vi "Main_copy.vi"(0 "PID On":bool) -> (5 "Total (V)":dbl[](array[slide]) scale=-8.0..8.0, 6 "Force (N)":T3(graph)={"M1 ref force"=20.0, "M2 ref force"=10.768311870905725, "M1 mes force"=3.690819426740976, "M2 mes force"=4.004504201458466})   [LabVIEW 2021]
uses:
  <vilib>/Platform/TimedLoop/XDataNode/timing_clust.ctl
  <vilib>/Platform/TimedLoop/XDataNode/nitl_modes.ctl
  <vilib>/Platform/TimedLoop/XDataNode/wakeup.ctl
  <vilib>/DAQmx/write.llb/DAQmx Write (Digital 1D Bool 1Chan 1Samp).vi
  <vilib>/DAQmx/write.llb/DAQmx Write (Analog 1D DBL NChan 1Samp).vi
  <vilib>/DAQmx/create/channels.llb/DAQmx Create Channel (DO-Digital Output).vi
  <vilib>/DAQmx/create/channels.llb/DAQmx Create Channel (AO-Voltage-Basic).vi
  <vilib>/DAQmx/create/channels.llb/DAQmx Create Channel (AI-Voltage-Basic).vi
  <vilib>/addons/control/pid/pid.llb/PID (DBL).vi
  <vilib>/DAQmx/miscellaneous.llb/DAQmx Fill In Error Info.vi
  <vilib>/Platform/TimedLoop/XDataNode/XDataNode.xnode
  <vilib>/Platform/TimedLoop/XDataNode/XDNodeRunTimeDep.lvlib
  <vilib>/addons/control/pid/NI_PID_pid.lvlib
panel:
  out "Control Time (ms)":i32
  out "Real Time (ms)":u32
  in  "RBF":bool
  in  "Traj Start":bool
  in  "PID gains":T1={"proportional gain (Kc)"=0.15, "integral time (Ti, min)"=0.0, "derivative time (Td, min)"=0.0} {"derivative time (Td, min)" format="%.3f"; "integral time (Ti, min)" format="%.3f"; "proportional gain (Kc)" format="%.3f"}
  out "output":dbl(slide)=-9.231688129094275 scale=-40.0..40.0
  in  "Set Tension":dbl=3.0
  in  "PID Tab":enum32{"PID Gain", "PIN On"}(tab)=enum."PIN On"
  in  "Gains":T2(array[cluster])=[{"proportional gain (Kc)"=0.17, "integral time (Ti, min)"=0.0, "derivative time (Td, min)"=0.0}, {"proportional gain (Kc)"=0.17, "integral time (Ti, min)"=0.0, "derivative time (Td, min)"=0.0}] {"derivative time (Td, min)" format="%.3f"; "integral time (Ti, min)" format="%.3f"; "proportional gain (Kc)" format="%.3f"}
  out "PID (V)":dbl[](array[slide])=[2.7725606974540344, 1.0] scale=-8.0..8.0
  out "Position (mm)":cluster{"Position":dbl, "ref_x (mm)":dbl}(graph)={"Position"=61.544587527295164, "ref_x (mm)"=0.0}
  in  "Loadcell":bool
  in  "Encoder":bool
  out "Speed (RPM)":dbl[](array[knob]) scale=-200.0..200.0
  out "time (s)":dbl=637.168
  in  "Set Point":dbl(slide)=19.690402476780186 scale=0.0..40.0
  in  "Motor Enable":bool[](array[boolean])=[FALSE, FALSE]
  in  "stop":bool
  # "FORCE"
  # "TRAJECTORY"
  # "INITIALIZE"
  # "TUNE"
  # "MONITOR"
  # "DEVEL"
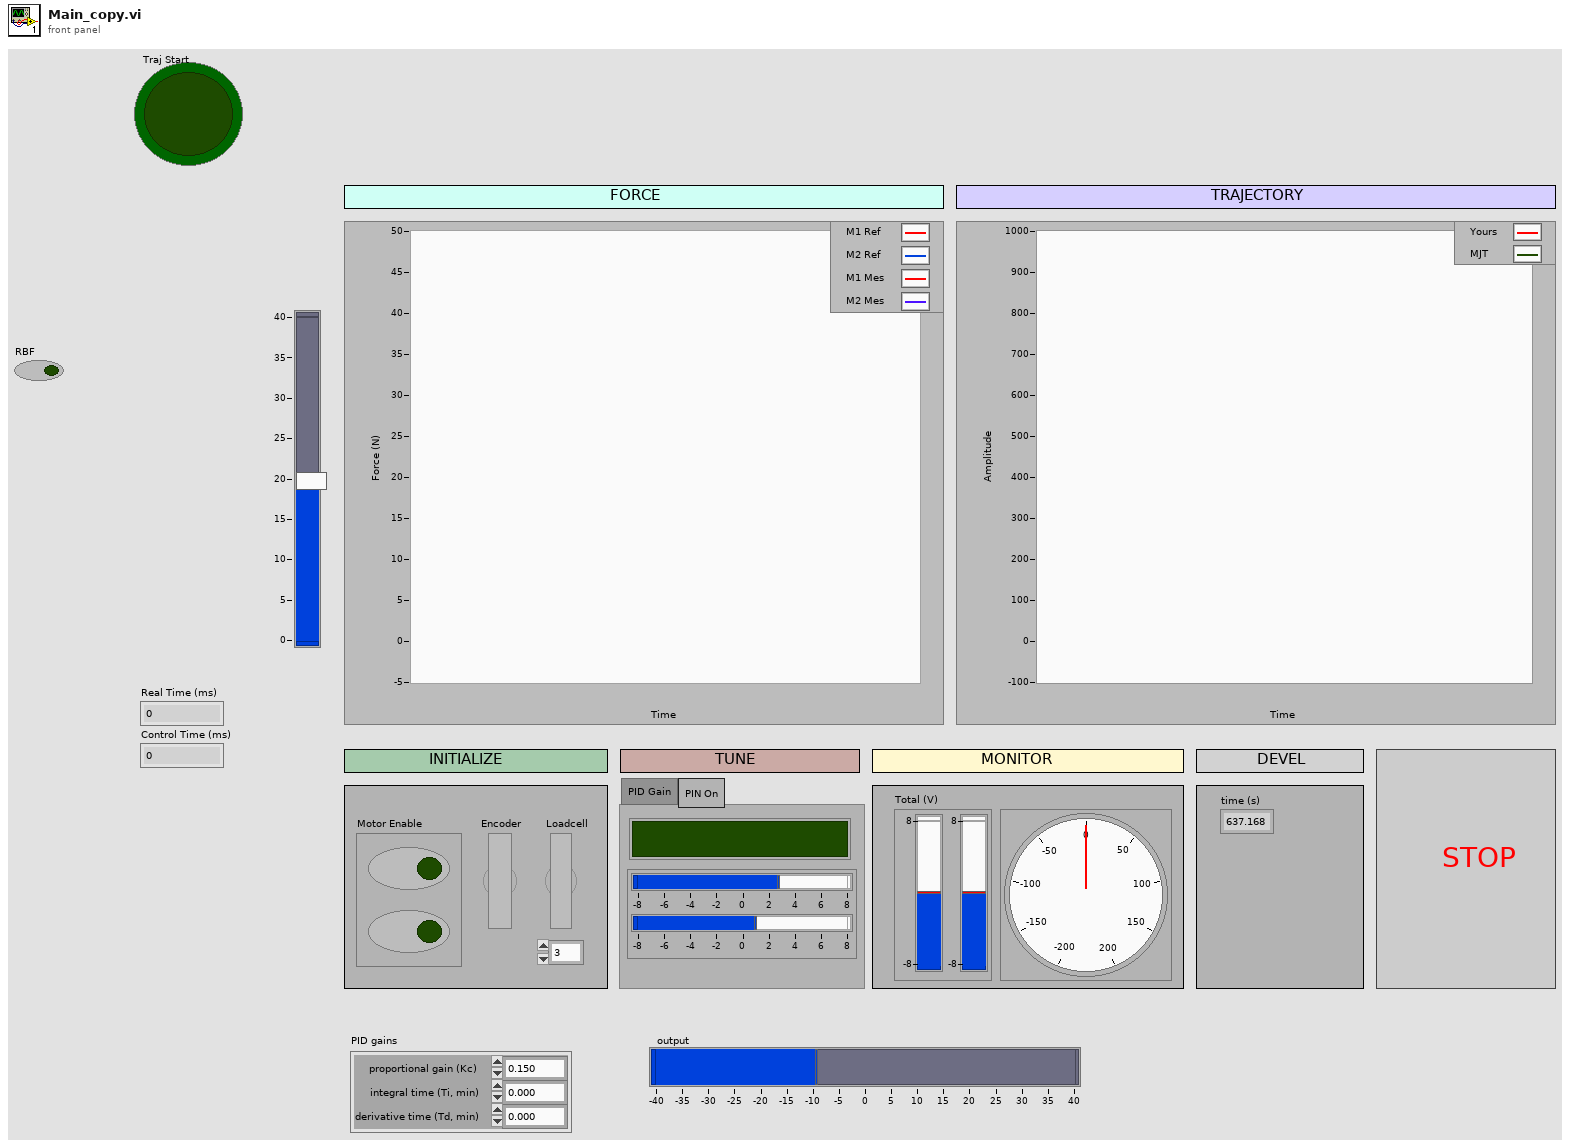
[diagram p1: front panel]
types:
  T1 = cluster{"proportional gain (Kc)":dbl, "integral time (Ti, min)":dbl, "derivative time (Td, min)":dbl}
  T2 = cluster{"proportional gain (Kc)":dbl, "integral time (Ti, min)":dbl, "derivative time (Td, min)":dbl}[]
  T3 = cluster{"M1 ref force":dbl, "M2 ref force":dbl, "M1 mes force":dbl, "M2 mes force":dbl}
  T4 = typedef "XDNodeRunTimeDep.lvlib/timing_clust.ctl" = cluster{"Expected End [f-1]":u64, "Actual End [f-1]":u64, "Finished Late? [f-1]":bool, "Expected End [i-1]":u64, "Actual End [i-1]":u64, "Finished Late? [i-1]":bool, "Expected Start [i]":u64, "Actual Start [i]":u64, "Expected Start [f]":u64, "Actual Start [f]":u64, "Source Name":string, "Structure Name":string, "Period":i64, "Deadline":i64, "Offset":i64, "Start":i64, "Priority":i32, "Timeout":i32, "Mode":T5, "Wakeup Reason":T6, "Error":errorcluster, "Source Type":string, "Secondary Source Type":string, "Global End Time":u64, "Global Start Time":u64, "Frame Duration":u64, "Iteration Duration":u64, "Assigned CPU":i32, "I/O Scan Engine Mode":u32}
  T5 = typedef "XDNodeRunTimeDep.lvlib/nitl_modes.ctl" = enum32{"No Change", "Process missed periods, maintain original phase", "Discard missed periods, maintain original phase", "Process missed periods, ignore original phase", "Discard missed periods, ignore original phase"}
  T6 = typedef "XDNodeRunTimeDep.lvlib/wakeup.ctl" = enum32{"Normal", "Aborted", "Asynchronous wakeup", "Timing source error", "Timed loop error", "Timeout"}
  T7 = cluster{"Total Time":dbl, "Total Length":dbl, "Control Freq":dbl}
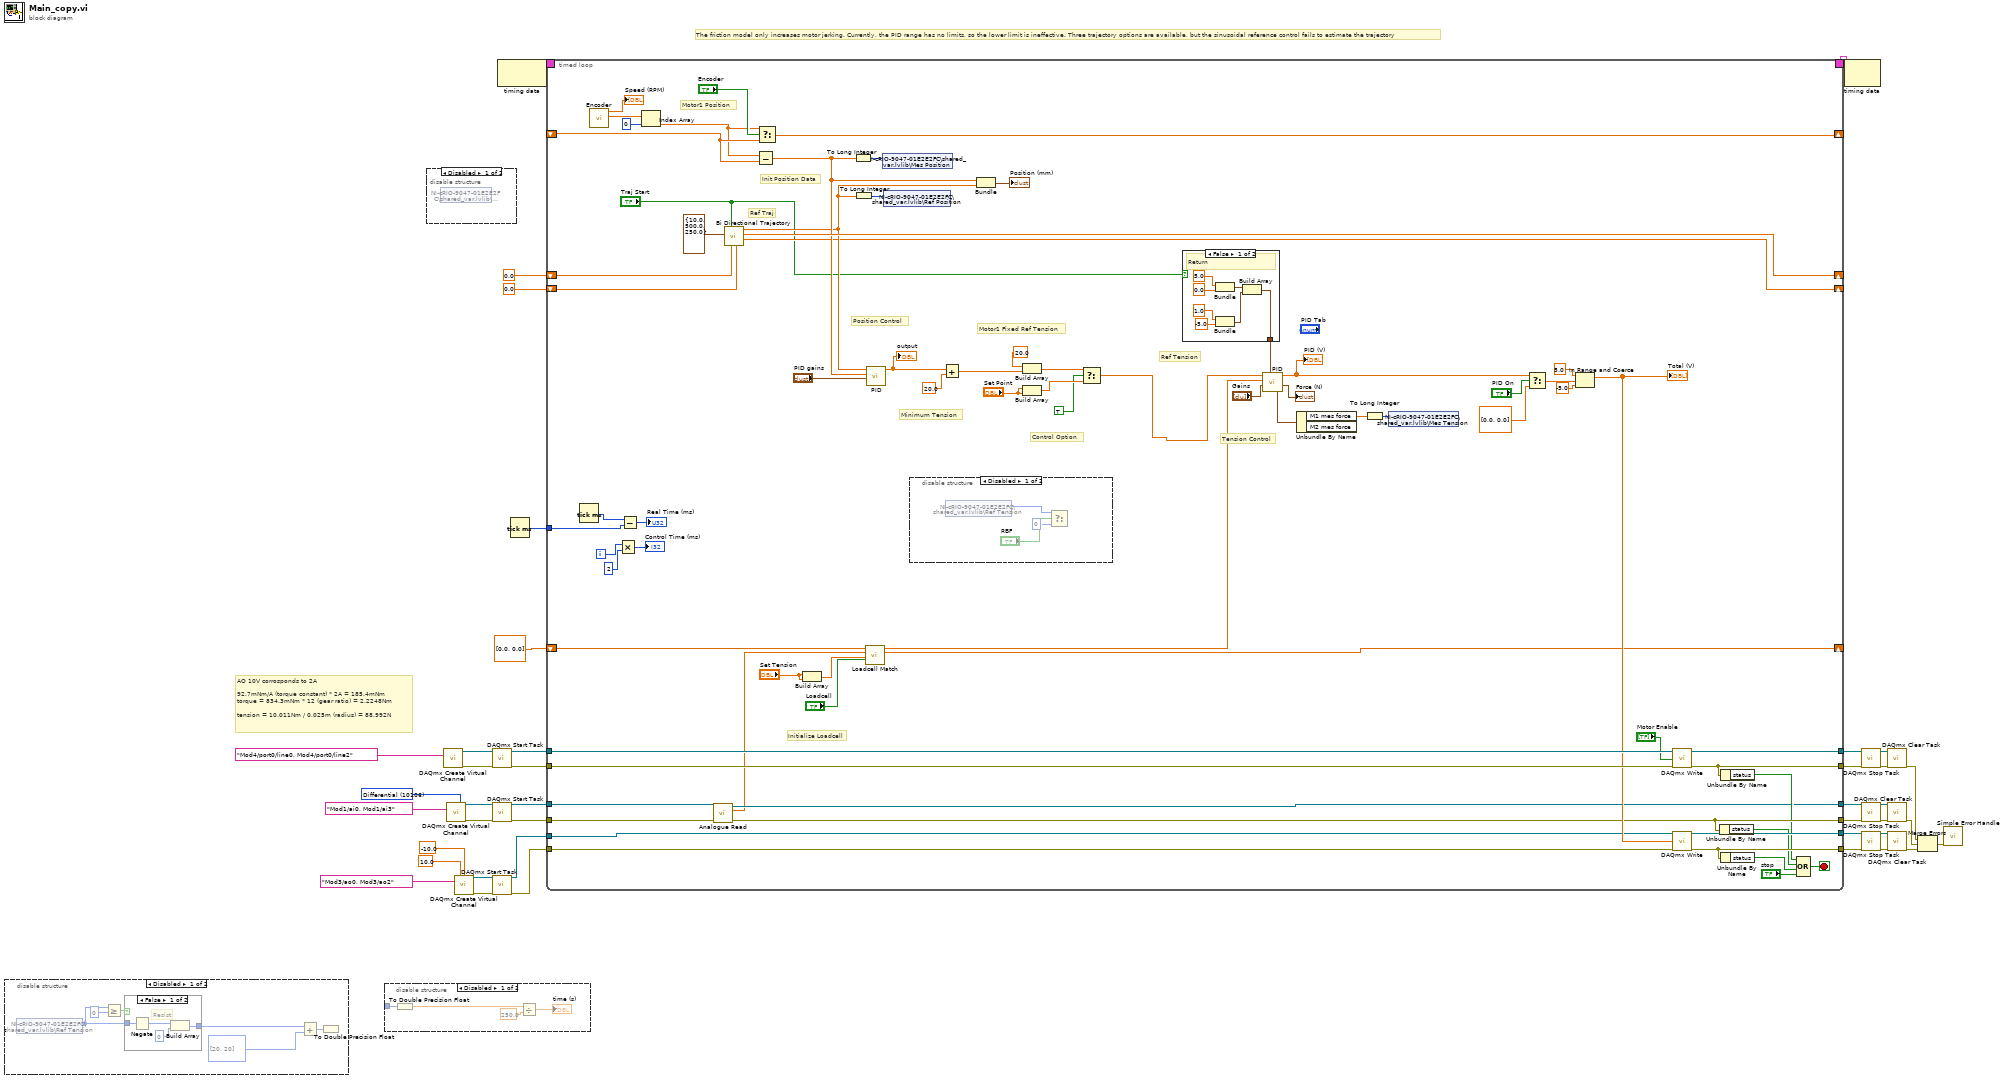
[diagram p0: block diagram]
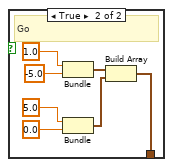
[diagram p3: hidden frame]
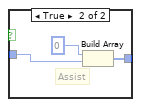
[diagram p6: hidden frame]
diagram:
  w5 = 10106 items=["Default"=-1, "RSE"=10083, "NRSE"=10078, "Differential"=10106, "Pseudodifferential"=12529] ("input terminal configuration")
  # "The friction model only increases motor jerking. Currently, the PID range has no limits, so the lower limit is ineffective. Three trajectory options are available, but the sinusoidal reference control fails to estimate the trajectory"
  # "AO 10V corrosponds to 2A\n\n92.7mNm/A (torque constant) * 2A = 185.4mNm\ntorque = 834.3mNm * 12 (gear ratio) = 2.2248Nm\n\ntension = 10.011Nm / 0.025m (radius) = 88.992N"
  n1 = disable-structure shown="Disabled" {
    frame Disabled {
      n2 = shared-variable "NI-cRIO-9047-01E2E2FC\\shared_var.lvlib\\Ref Tension"() -> (w43:i32)  [unwired: 1 in, 1 out]
      n3 = Greater Or Equal?(x=w43, y=0) -> (x >= y?=w41:bool)
      n4 = case shown="False" w41 {
        tunnel: w43 -> [w49 w52]
        tunnel: [w50 w53] -> w46
        frame False {
          # "Resist"
          n5 = Negate(x=w49) -> (-x=w47:i32)
          n6 = Build Array(w47, 0 ("element")) -> (w50:i32[])
        }
        frame True {
          # "Assist"
          n7 = Build Array(0 ("element"), w52) -> (w53:i32[])
        }
      }
      n8 = Add(x=w46, y=i32[] [20, 20] ("x")) -> (x+y=w44:i32[])
      n9 = To Double Precision Float(number=w44) -> ()  [unwired: 1 out]
    }
    frame Enabled {
    }
  }
  n10 = disable-structure shown="Disabled" {
    disable-tunnel: _ -> [w57 _]
    frame Disabled {
      n11 = To Double Precision Float(number=w57) -> (double precision float=w56:dbl)
      n12 = Divide(x=w56, y=250.0) -> (x/y=→"time (s)":dbl)
    }
    frame Enabled {
    }
  }
  n13 = disable-structure shown="Disabled" {
    frame Disabled {
      n14 = shared-variable "NI-cRIO-9047-01E2E2FC\\shared_var.lvlib\\Trigger"() -> ()  [unwired: 1 in, 2 out]
    }
    frame Enabled {
    }
  }
  n15 = call-poly <vilib>:"DAQmx Create Virtual Channel.vi"("lines"=tag "Mod4/port0/line0, Mod4/port0/line2") -> ("task out"=w32:refnum<k21>, "error out"=w31:errorcluster)  [unwired: 13 in]
  n16 = call-poly <vilib>:"DAQmx Create Virtual Channel.vi"("input terminal configuration"=w5, "physical channels"=tag "Mod1/ai0, Mod1/ai3") -> ("task out"=w22:refnum<k21>, "error out"=w23:errorcluster)  [unwired: 12 in]
  n17 = call-poly <vilib>:"DAQmx Create Virtual Channel.vi"("maximum value"=10.0 ("AO max"), "minimum value"=-10.0 ("AO min"), "physical channels"=tag "Mod3/ao0, Mod3/ao2" ("Physical Channel(s)")) -> ("task out"=w16:refnum<k21>, "error out"=w15:errorcluster)  [unwired: 11 in]
  n18 = call <vilib>:"DAQmx Start Task.vi"("task/channels in"=w32, "error in"=w31) -> ("task out"=w29:refnum<k21>, "error out"=w28:errorcluster)  [unwired: 12 in]
  n19 = call <vilib>:"DAQmx Start Task.vi"("task/channels in"=w22, "error in"=w23) -> ("task out"=w20:refnum<k21>, "error out"=w19:errorcluster)  [unwired: 12 in]
  n20 = call <vilib>:"DAQmx Start Task.vi"("task/channels in"=w16, "error in"=w15) -> ("task out"=w34:refnum<k21>, "error out"=w33:errorcluster)  [unwired: 12 in]
  n21 = node-c288() -> (w36:T4)  [unwired: 1 in]
  n22 = Tick Count (ms)() -> (millisecond timer value=w1:u32)
  n23 = timed-loop {
    tunnel: [w128] -> w40
    tunnel: [w127] -> w39
    tunnel: [w92] -> w38
    tunnel: [w114] -> w37
    tunnel: w20 -> [w125]
    timing: w36 -> [_]
    timing-out: [_] -> w35
    tunnel: w19 -> [w124]
    tunnel: w34 -> [w91]
    tunnel: w33 -> [w126]
    tunnel: w29 -> [w123]
    tunnel: w28 -> [w122]
    tunnel: [w121] -> w25
    tunnel: [w115] -> w24
    shift-right: [w100] -> _
    shift-left: 0.0 ("total time") -> [w101]
    shift-right: [w95] -> _
    shift-left: _ -> [w93]
    shift-right: [w85] -> _
    shift-left: dbl[] [0.0, 0.0] ("measured force") -> [w86]
    shift-right: [w73] -> _
    shift-left: 0.0 ("total time") -> [w74]
    tunnel: w1 -> [w61]
    i -> [w64]
    stop <- w110 stop-if-true
    # "Initialize Loadcell"
    # "Tension Control"
    # "Ref Tension"
    # "Position Control"
    # "Ref Traj"
    # "Control Option"
    # "Motor1 Fixed Ref Tension"
    # "Minimum Tension"
    # "Init Position Data"
    # "Motor1 Position"
    n24 = Tick Count (ms)() -> (millisecond timer value=w62:u32)
    n25 = call "Encoder.vi"() -> ("Mes Pos (mm)"=w98:dbl[], "RPM"=→"Speed (RPM)":dbl[])  [unwired: 10 in]
    n26 = Multiply(x=w64, y=2) -> (x*y=→"Control Time (ms)":i32)
    n27 = Subtract(x=w62, y=w61) -> (x-y=→"Real Time (ms)":u32)
    n28 = Index Array(array=w98, index=0) -> (element=w67:dbl)
    n29 = call "Analogue Read.vi"("error in"=w124, "task/channels in"=w125) -> ("error out"=w114:errorcluster, "measured force"=w83:dbl[], "task out"=w92:refnum<k21>)  [unwired: 6 in, 1 out]
    n30 = call "Bi Directional Trajectory.vi"("Return Time"=w74, "Go Time"=w101, "Traj Start"="Traj Start", "Trajectory Settings"=T7 {"Total Time"=10.0, "Total Length"=500.0, "Control Freq"=250.0}) -> ("Return Next Time"=w73:dbl, "Go Next Time"=w100:dbl, "Output (mm)"=w76:dbl)  [unwired: 5 in]
    n31 = Subtract(x=w67, y=w93) -> (x-y=w77:dbl)
    n32 = Select(t=w67, s="Encoder", f=w93) -> (s? t:f=w95:dbl)
    n33 = Build Array("Set Tension", "Set Tension") -> (w78:dbl[])
    n34 = To Long Integer(number=w77) -> (32bit integer=w81:i32)
    n35 = To Long Integer(number=w76) -> (32bit integer=w82:i32)
    n36 = call "Loadcell Match.vi"("Initialize"="Loadcell", "Set Tension"=w78, "Mes Tension"=w83, "Next Tension Error"=w86) -> ("Tension Error"=w85:dbl[], "Filtered Tension"=w84:dbl[])  [unwired: 6 in]
    n37 = call-poly <vilib>:"PID.vi"("PID gains"="PID gains", "process variable"=w77, "setpoint"=w76) -> ("output"=w70:dbl)  [unwired: 7 in, 1 out]
    "output" <- w70
    n38 = shared-variable "NI-cRIO-9047-01E2E2FC\\shared_var.lvlib\\Mes Position"(w81) -> ()  [unwired: 1 in, 1 out]
    n39 = shared-variable "NI-cRIO-9047-01E2E2FC\\shared_var.lvlib\\Ref Position"(w82) -> ()  [unwired: 1 in, 1 out]
    n40 = disable-structure shown="Disabled" {
      frame Disabled {
        n41 = shared-variable "NI-cRIO-9047-01E2E2FC\\shared_var.lvlib\\Ref Tension"() -> (w131:i32)  [unwired: 1 in, 1 out]
        n42 = Select(t=w131, s="RBF", f=0) -> ()  [unwired: 1 out]
      }
      frame Enabled {
      }
    }
    n43 = Add(x=w70, y=20.0) -> (x+y=w69:dbl)
    n44 = Bundle(w77, "Output (mm)"=w76) -> (→"Position (mm)":cluster{dbl, "Output (mm)":dbl})  [unwired: 1 in]
    n45 = Build Array(20.0 ("element"), w69) -> (w68:dbl[])
    n46 = Build Array("Set Point", "Set Point") -> (w104:dbl[])
    n47 = Select(t=w68, s=TRUE, f=w104) -> (s? t:f=w58:dbl[])
    n48 = case shown="False" "Traj Start" {
      tunnel: [w132 w139] -> w88
      frame False {
        # "Return"
        n49 = Bundle(5.0, 0.0) -> (w138:cluster{dbl, dbl})  [unwired: 1 in]
        n50 = Bundle(1.0, -5.0) -> (w137:cluster{dbl, dbl})  [unwired: 1 in]
        n51 = Build Array(w138, w137) -> (w132:cluster{dbl, dbl}[])
      }
      frame True {
        # "Go"
        n52 = Bundle(1.0, -5.0) -> (w140:cluster{dbl, dbl})  [unwired: 1 in]
        n53 = Bundle(5.0, 0.0) -> (w141:cluster{dbl, dbl})  [unwired: 1 in]
        n54 = Build Array(w140, w141) -> (w139:cluster{dbl, dbl}[])
      }
    }
    n55 = call <vilib>:"PID.vi"("output range"=w88, "PID gains"="Gains", "mes force"=w84, "ref force"=w58) -> ("output cluster"=w80:T3, "PID output"=w108:dbl[])  [unwired: 6 in]
    "Force (N)" <- w80
    "PID (V)" <- w108
    n56 = Unbundle By Name(w80) -> ("M1 mes force"=w89:dbl)  [unwired: 1 out]
    n57 = To Long Integer(number=w89) -> (32bit integer=w90:i32)
    n58 = shared-variable "NI-cRIO-9047-01E2E2FC\\shared_var.lvlib\\Mes Tension"(w90) -> ()  [unwired: 1 in, 1 out]
    n59 = Select(t=w108, s="PID On", f=dbl[] [0.0, 0.0]) -> (s? t:f=w106:dbl[])
    n60 = In Range and Coerce(upper limit=5.0, x=w106, lower limit=-5.0) -> (coerced(x)=w116:dbl[])  [unwired: 1 out]
    "Total (V)" <- w116
    n61 = call-poly <vilib>:"DAQmx Write.vi"("task/channels in"=w123, "data"="Motor Enable", "error in"=w122) -> ("task out"=w121:refnum<k21>, "error out"=w115:errorcluster)  [unwired: 10 in, 1 out]
    n62 = call-poly <vilib>:"DAQmx Write.vi"("task/channels in"=w91, "data"=w116, "error in"=w126) -> ("task out"=w128:refnum<k21>, "error out"=w127:errorcluster)  [unwired: 10 in, 1 out]
    n63 = Unbundle By Name(w114) -> ("status"=w112:bool)
    n64 = Unbundle By Name(w115) -> ("status"=w111:bool)
    n65 = Unbundle By Name(w127) -> ("status"=w113:bool)
    n66 = Compound Arithmetic op=OR(w111, w112, w113, "stop") -> (w110:bool)
  }
  n67 = node-c288(w35) -> ()  [unwired: 1 out]
  n68 = call <vilib>:"DAQmx Stop Task.vi"("task/channels in"=w25, "error in"=w24) -> ("task out"=w27:refnum<k21>, "error out"=w26:errorcluster)  [unwired: 12 in]
  n69 = call <vilib>:"DAQmx Stop Task.vi"("task/channels in"=w38, "error in"=w37) -> ("task out"=w11:refnum<k21>, "error out"=w10:errorcluster)  [unwired: 12 in]
  n70 = call <vilib>:"DAQmx Stop Task.vi"("task/channels in"=w40, "error in"=w39) -> ("task out"=w13:refnum<k21>, "error out"=w12:errorcluster)  [unwired: 12 in]
  n71 = call <vilib>:"DAQmx Clear Task.vi"("task in"=w27, "error in"=w26) -> ("error out"=w6:errorcluster)  [unwired: 13 in]
  n72 = call <vilib>:"DAQmx Clear Task.vi"("task in"=w11, "error in"=w10) -> ("error out"=w7:errorcluster)  [unwired: 13 in]
  n73 = call <vilib>:"DAQmx Clear Task.vi"("task in"=w13, "error in"=w12) -> ("error out"=w8:errorcluster)  [unwired: 13 in]
  n74 = Merge Errors(w6, w7, w8) -> (w9:errorcluster)
  n75 = call <vilib>:"Simple Error Handler.vi"("error in (no error)"=w9) -> ()  [unwired: 4 in, 5 out]
